vi "Start Test.vi"(8 "error in (no error)":errorcluster, 10 "Selected Tests":string[](array[string]), 11 "Test Application Controller in":refnum<class "Test Application Controller.lvclass">) -> (0 "error out":errorcluster, 3 "Test Application Controller out":refnum<class "Test Application Controller.lvclass">)   [LabVIEW 2017, in "Test Application Controller.lvlib" / "Test Application Controller.lvclass"]
uses:
  Test Application Controller.lvclass
  Test Application Controller.lvclass/Test Application Controller.ctl
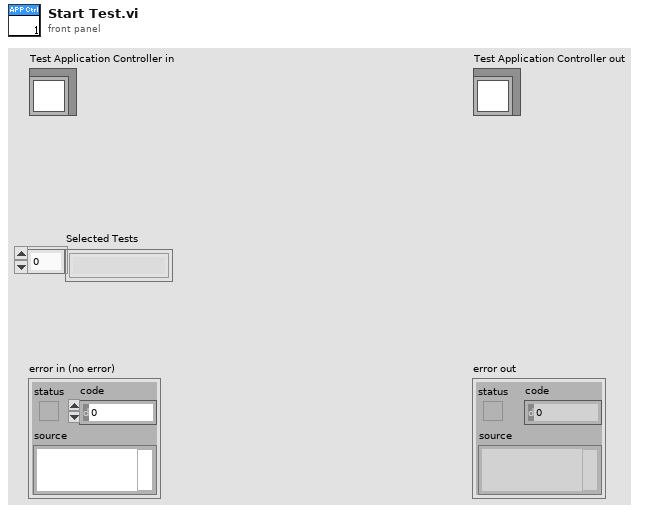
[diagram p1: front panel]
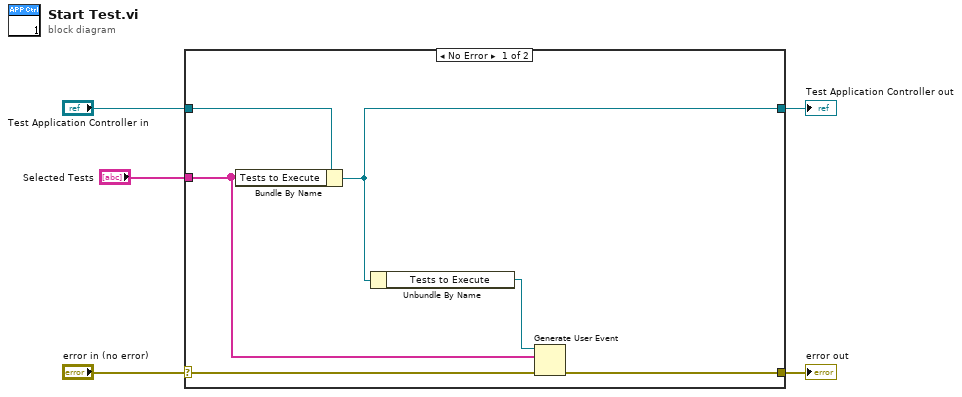
[diagram p0: block diagram]
diagram:
  n1 = case shown="No Error" "error in (no error)" {
    selector: "error in (no error)" -> [w8 w13]
    tunnel: [w7 w13] -> w4
    tunnel: [w10 w12] -> w2
    tunnel: "Test Application Controller in" -> [w11 w12]
    tunnel: "Selected Tests" -> [w6 _]
    frame No Error {
      n2 = Bundle By Name(cluster=w11, "Tests to Execute"=w6) -> (w10:refnum<class "Test Application Controller.lvclass">)
      n3 = Unbundle By Name(w10) -> ("Tests to Execute"=w9:refnum<user-event>)
      n4 = Generate User Event(user event=w9, event data cluster=w6, error in=w8) -> (error out=w7:errorcluster)  [unwired: 1 in, 1 out]
    }
    frame Error {
    }
  }
  "error out" <- w4
  "Test Application Controller out" <- w2
